vi "Variant_CreateEmptyNestedCluster.vi"(7 "Separator (dot)":string, 11 "Namespaced Cluster":string) -> (3 "Empty Nested Cluster":variant)   [LabVIEW 2013, in "OpenVariant.lvlib"]
uses:
  OpenVariant.lvlib
  <vilib>/Utility/GetType.llb/TD_Create Cluster.vi
  Conversions/OpenConvert.lvlib
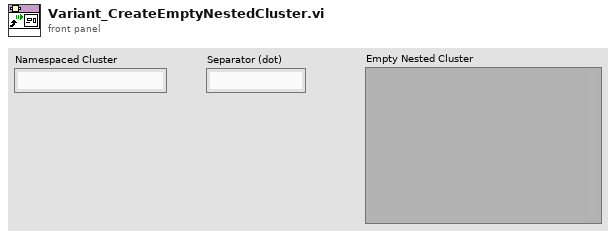
[diagram p1: front panel]
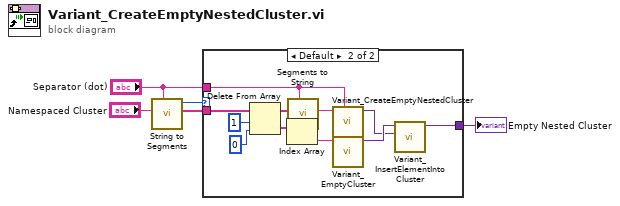
[diagram p0: block diagram]
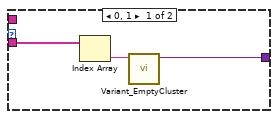
[diagram p2: hidden frame]
diagram:
  n1 = call "String to Segments.vi"("Separator (dot)"="Separator (dot)", "String"="Namespaced Cluster") -> ("Segments"=w4:string[], "Nb segments"=w3:i32)  [unwired: 8 in]
  n2 = case shown="Default" w3 {
    tunnel: w4 -> [w7 w19]
    tunnel: [w8 w10] -> w2
    tunnel: "Separator (dot)" -> [_ w18]
    frame 0, 1 {
      n3 = Index Array(array=w7) -> (element=w6:string)  [unwired: 1 in]
      n4 = call "Variant_EmptyCluster.vi"("Cluster Name"=w6) -> ("Empty Cluster"=w8:variant)  [unwired: 10 in]
    }
    frame Default {
      n5 = Delete From Array(array=w19, length=1, index=0) -> (deleted portion=w16:string[], array with subset deleted=w15:string[])
      n6 = Index Array(array=w16) -> (element=w13:string)  [unwired: 1 in]
      n7 = call "Segments to String.vi"("Separator (dot)"=w18, "Segments"=w15) -> ("String"=w14:string)  [unwired: 9 in]
      n8 = call "Variant_CreateEmptyNestedCluster.vi"("Separator (dot)"=w18, "Namespaced Cluster"=w14) -> ("Empty Nested Cluster"=w11:variant)  [unwired: 9 in]
      n9 = call "Variant_EmptyCluster.vi"("Cluster Name"=w13) -> ("Empty Cluster"=w12:variant)  [unwired: 10 in]
      n10 = call "Variant_InsertElementIntoCluster.vi"("Element"=w11, "Cluster in"=w12) -> ("Cluster out"=w10:variant)  [unwired: 9 in]
    }
  }
  "Empty Nested Cluster" <- w2
